vi "ExtensionLogic.vi"   [LabVIEW 2020]
uses:
  Robot Global Data.vi
  Swerve Global Variables.vi
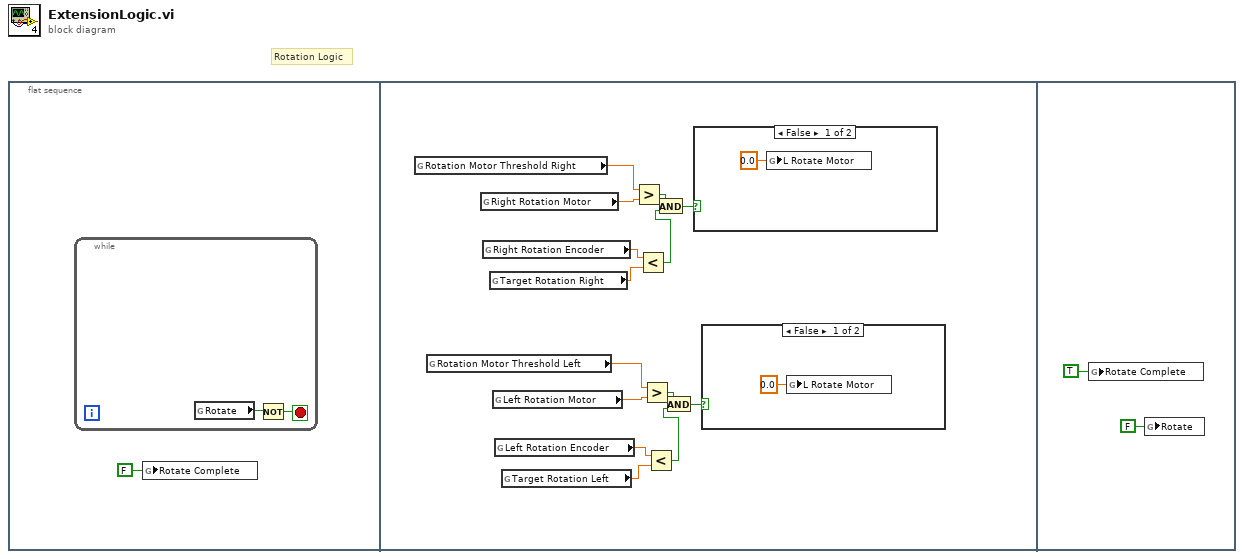
[diagram p0: block diagram]
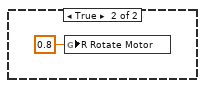
[diagram p2: hidden frame]
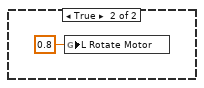
[diagram p3: hidden frame]
diagram:
  # "Rotation Logic"
  n1 = flat-sequence {
    frame #0 {
      n2 = while {
        stop <- w2 stop-if-true
        n3 = global read "Robot Global Data.vi" "Rotate"() -> (w3:bool)
        n4 = Not(x=w3) -> (.not. x?=w2:bool)
      }
      n5 = global write "Robot Global Data.vi" "Rotate Complete"(FALSE ("Extend Complete")) -> ()
    }
    frame #1 {
      n6 = global read "Swerve Global Variables.vi" "Rotation Motor Threshold Right"() -> (w6:dbl)
      n7 = global read "Swerve Global Variables.vi" "Rotation Motor Threshold Left"() -> (w13:dbl)
      n8 = global read "Swerve Global Variables.vi" "Right Rotation Motor"() -> (w5:dbl)
      n9 = global read "Swerve Global Variables.vi" "Right Rotation Encoder"() -> (w9:dbl)
      n10 = global read "Swerve Global Variables.vi" "Target Rotation Right"() -> (w8:dbl)
      n11 = global read "Swerve Global Variables.vi" "Left Rotation Motor"() -> (w12:dbl)
      n12 = global read "Swerve Global Variables.vi" "Left Rotation Encoder"() -> (w16:dbl)
      n13 = global read "Swerve Global Variables.vi" "Target Rotation Left"() -> (w15:dbl)
      n14 = Greater?(x=w6, y=w5) -> (0:w4:bool)
      n15 = Less?(x=w9, y=w8) -> (x < y?=w7:bool)
      n16 = Greater?(x=w13, y=w12) -> (0:w11:bool)
      n17 = Less?(x=w16, y=w15) -> (x < y?=w14:bool)
      n18 = And(x=w4, y=w7) -> (x .and. y?=w10:bool)
      n19 = And(x=w11, y=w14) -> (x .and. y?=w17:bool)
      n20 = case shown="False" w10 {
        frame False {
          n21 = global write "Swerve Global Variables.vi" "L Rotate Motor"(0.0 ("L Rotate Motor")) -> ()
        }
        frame True {
          n22 = global write "Swerve Global Variables.vi" "R Rotate Motor"(0.8 ("L Rotate Motor")) -> ()
        }
      }
      n23 = case shown="False" w17 {
        frame False {
          n24 = global write "Swerve Global Variables.vi" "L Rotate Motor"(0.0 ("L Rotate Motor")) -> ()
        }
        frame True {
          n25 = global write "Swerve Global Variables.vi" "L Rotate Motor"(0.8 ("L Rotate Motor")) -> ()
        }
      }
    }
    frame #2 {
      n26 = global write "Robot Global Data.vi" "Rotate Complete"(TRUE ("Extend Complete")) -> ()
      n27 = global write "Robot Global Data.vi" "Rotate"(FALSE ("Rotate")) -> ()
    }
  }
